vi "Create Action.vi"(8 "error in (no error)":errorcluster, 10 "State":T1, 11 "BangBangControl in":refnum<class "BangBangControl.lvclass">) -> (0 "error out":errorcluster, 2 "Action":T2, 3 "BangBangControl out":refnum<class "BangBangControl.lvclass">)   [LabVIEW 2020, in "VolatusControl.lvlib" / "BangBangControl.lvclass"]
uses:
  BangBangControl.lvclass
  BangBangControl.lvclass/BangBangControl.ctl
  Volatus/MessageQ/MessageQ.lvclass
  Valve Action.ctl
  VolatusControl.lvlib
  State.ctl
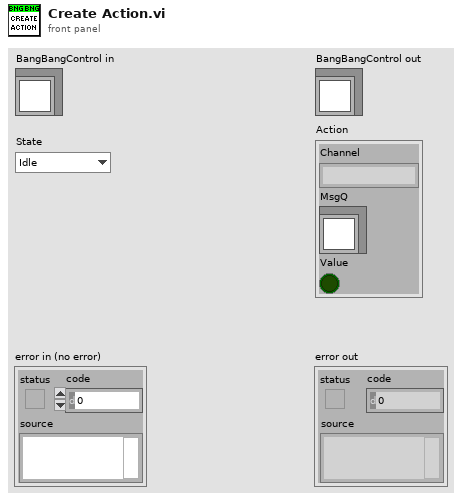
[diagram p1: front panel]
types:
  T1 = typedef "VolatusControl.lvlib/BangBangControl.lvclass/State.ctl" = enum16{"Idle", "RampUp", "RampDown", "Hold", "Disable", "Enable"}
  T2 = typedef "VolatusControl.lvlib/Valve Action.ctl" = cluster{"Channel":string, "MsgQ":refnum<class "MessageQ.lvclass">, "Value":bool}
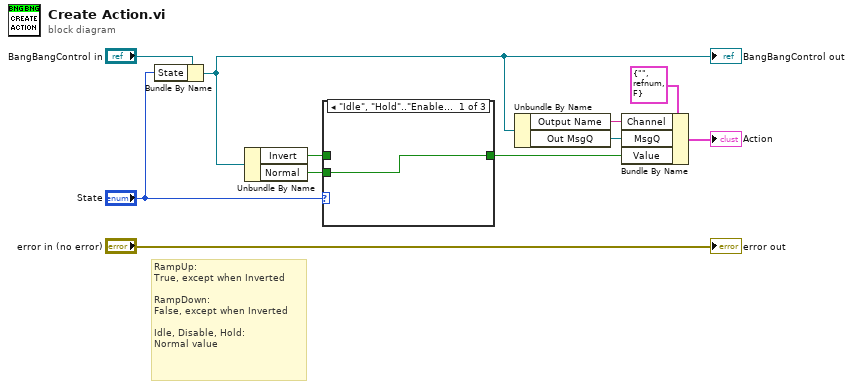
[diagram p0: block diagram]
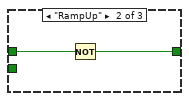
[diagram p2: hidden frame]
diagram:
  # "RampUp:\nTrue, except when Inverted\n\nRampDown:\nFalse, except when Inverted\n\nIdle, Disable, Hold:\nNormal value"
  n1 = Bundle By Name(cluster="BangBangControl in", "State"="State") -> (w4:refnum<class "BangBangControl.lvclass">)
  "BangBangControl out" <- w4
  n2 = Unbundle By Name(w4) -> ("Invert"=w8:bool, "Normal"=w7:bool)
  n3 = case shown="\"Idle\", \"Hold\"..\"Enable\"" "State" {
    tunnel: w8 -> [_ w14 w15]
    tunnel: w7 -> [w12 _ _]
    tunnel: [w12 w13 w15] -> w1
    frame "Idle", "Hold".."Enable" {
    }
    frame "RampUp" {
      n4 = Not(x=w14) -> (.not. x?=w13:bool)
    }
    frame "RampDown" {
    }
  }
  n5 = Unbundle By Name(w4) -> ("Output Name"=w3:string, "Out MsgQ"=w2:refnum<class "MessageQ.lvclass">)
  n6 = Bundle By Name(cluster=T2 {"Channel"="", "MsgQ"=refnum, "Value"=FALSE} ("Action"), "Channel"=w3, "MsgQ"=w2, "Value"=w1) -> (→"Action":T2)
  "error out" <- "error in (no error)"
